vi "register child.vi"(8 "error in":errorcluster, 10 "child":refnum<class "communicator.lvclass">, 11 "communicator in":refnum<class "communicator.lvclass">) -> (0 "error out":errorcluster, 3 "communicator out":refnum<class "communicator.lvclass">)   [LabVIEW 2015, in "communicator.lvclass"]
uses:
  communicator.lvclass
  communicator.lvclass/communicator.ctl
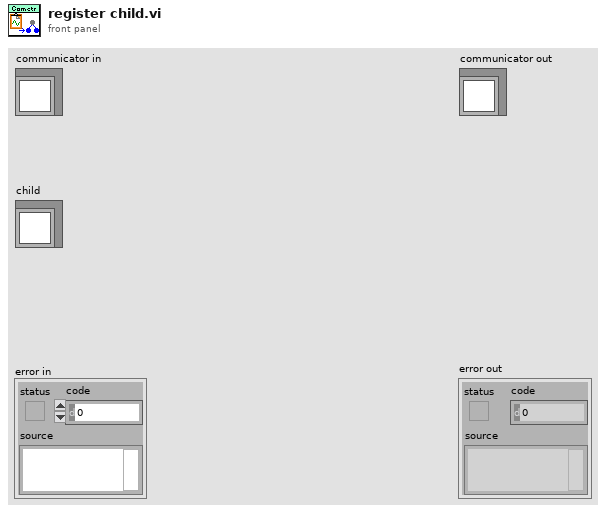
[diagram p1: front panel]
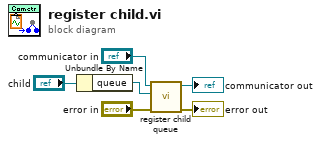
[diagram p0: block diagram]
diagram:
  n1 = Unbundle By Name("child") -> ("queue"=w1:refnum<class "identifying queue.lvclass">)
  n2 = call "register child queue.vi"("error in"="error in", "queue"=w1, "communicator in"="communicator in") -> ("error out"=→"error out":errorcluster, "communicator out"=→"communicator out":refnum<class "communicator.lvclass">)  [unwired: 7 in]
